vi "实验5_3.vi"() -> ()   [LabVIEW 2018]
uses:
  <vilib>/Utility/file.llb/Write Delimited Spreadsheet (DBL).vi
  <vilib>/Utility/file.llb/Read Delimited Spreadsheet (DBL).vi
  <vilib>/Analysis/NI_AALBase.lvlib
panel:
  out "Array 2":cluster{"Array":dbl[]}[](array[cluster])
  out "Array 3":dbl[][](array[numeric])
  in  "Numeric":dbl=20.0
  in  "Path":path=path "/Users/fancheyv/Desktop/大三下实验/LabView/file"
  out "Array":dbl[][](array[numeric])
  out "Waveform Graph 3":dbl[][](graph)
  out "Waveform Graph 2":cluster{"Sinusoidal Pattern":dbl[]}[](graph)
  out "Waveform Graph":dbl[][](graph)
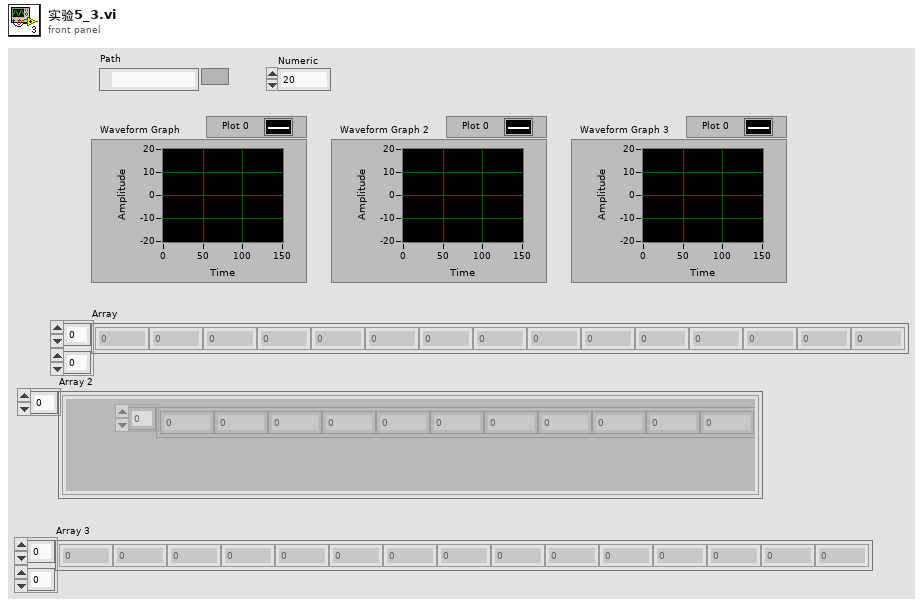
[diagram p1: front panel]
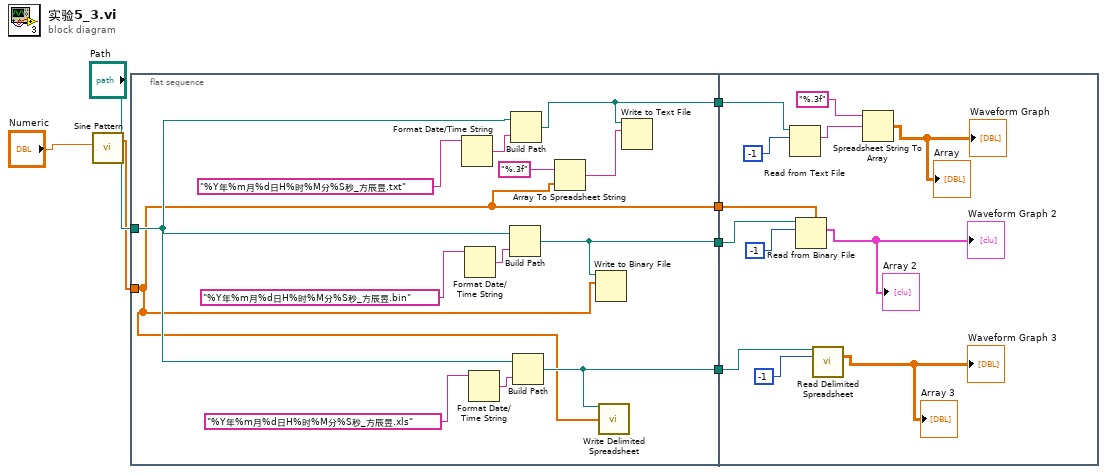
[diagram p0: block diagram]
diagram:
  n1 = call <vilib>:"Sine Pattern.vi"("amplitude"="Numeric") -> ("Sinusoidal Pattern"=w5:dbl[])  [unwired: 3 in, 1 out]
  n2 = flat-sequence {
    tunnel: "Path" -> [w14]
    tunnel: w5 -> [w8]
    tunnel: [w11] -> w4
    tunnel: [w10] -> w3
    tunnel: [w9] -> w2
    tunnel: [w8] -> w1
    tunnel: w4 -> [w28]
    tunnel: w3 -> [w29]
    tunnel: w2 -> [w30]
    tunnel: w1 -> [w26]
    frame #0 {
      n3 = Format Date/Time String(time format string (%c)="%Y年%m月%d日H%时%M分%S秒_方辰昱.txt") -> (date/time string=w17:string)  [unwired: 2 in]
      n4 = Format Date/Time String(time format string (%c)="%Y年%m月%d日H%时%M分%S秒_方辰昱.bin") -> (date/time string=w15:string)  [unwired: 2 in]
      n5 = Format Date/Time String(time format string (%c)="%Y年%m月%d日H%时%M分%S秒_方辰昱.xls") -> (date/time string=w16:string)  [unwired: 2 in]
      n6 = Build Path(base path=w14, name or relative path=w15) -> (appended path=w10:path)
      n7 = Build Path(base path=w14, name or relative path=w17) -> (appended path=w11:path)
      n8 = Build Path(base path=w14, name or relative path=w16) -> (appended path=w9:path)
      n9 = Array To Spreadsheet String(array=w8, 3:"%.3f") -> (spreadsheet string=w12:string)  [unwired: 1 in]
      n10 = Write to Binary File(file (use dialog)=w10, data=w8) -> ()  [unwired: 4 in, 3 out]
      n11 = call-poly <vilib>:"Write Delimited Spreadsheet.vi"("file path (dialog if empty)"=w9, "1D data"=w8) -> ()  [unwired: 12 in, 2 out]
      n12 = Write to Text File(file (use dialog)=w11, text=w12) -> ()  [unwired: 2 in, 3 out]
    }
    frame #1 {
      n13 = Read from Text File(file (use dialog)=w28, count=-1) -> (text=w24:string)  [unwired: 2 in, 3 out]
      n14 = Read from Binary File(5:w26, 10:-1, 11:w29) -> (2:→"Waveform Graph 2" →"Array 2":cluster{"Sinusoidal Pattern":dbl[]}[])  [unwired: 3 in, 3 out]
      n15 = call-poly <vilib>:"Read Delimited Spreadsheet.vi"("file path (dialog if empty)"=w30, "number of rows (all:-1)"=-1) -> ("all rows"=→"Waveform Graph 3" →"Array 3":dbl[][])  [unwired: 8 in, 5 out]
      n16 = Spreadsheet String To Array(format string="%.3f", spreadsheet string=w24) -> (array=→"Waveform Graph" →"Array":dbl[][])  [unwired: 2 in]
    }
  }
